vi "Read CamName and ImageType.vi"(8 "error in (no error)":errorcluster, 11 "IMAQdx Cam in":refnum<class "IMAQdx Cam.lvclass">) -> (0 "error out":errorcluster, 1 "Camera":T1, 2 "Image Type":T2 items=["Grayscale (U8)", "Grayscale (I16)", "Grayscale (SGL)", "Complex (CSG)", "RGB (U32)", "HSL (U32)", "RGB (U64)", "Grayscale (U16)"], 3 "IMAQdx Cam out":refnum<class "IMAQdx Cam.lvclass">)   [LabVIEW 2009, in "IMAQdx Cam.lvclass"]
uses:
  IMAQdx Cam.lvclass
  <vilib>/userDefined/High Color/IMAQdx.ctl
  IMAQdx Cam.lvclass/IMAQdx Cam.ctl
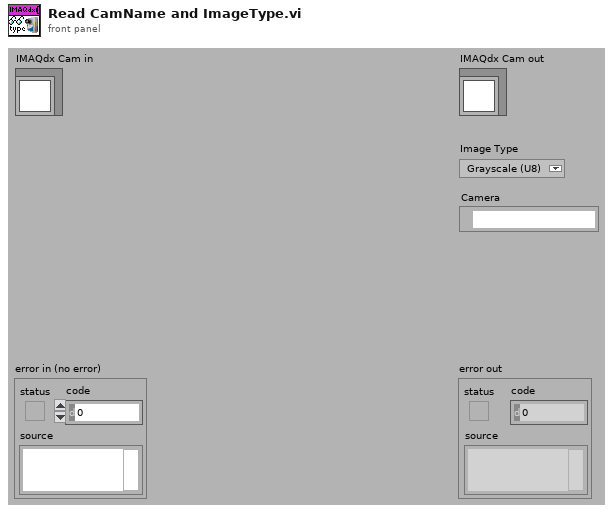
[diagram p1: front panel]
types:
  T1 = typedef "IMAQdx.ctl" = refnum<k21>
  T2 = typedef "Image Type" = u32
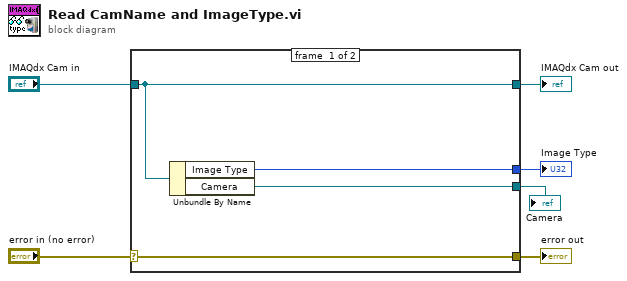
[diagram p0: block diagram]
diagram:
  n1 = case shown="No Error" "error in (no error)" {
    selector: "error in (no error)" -> [w10 w11]
    tunnel: [w10 w11] -> w5
    tunnel: [w9 w12] -> w3
    tunnel: "IMAQdx Cam in" -> [w9 w12]
    tunnel: [w8 _] -> w2
    tunnel: [w7 _] -> w1
    frame #0 {
      n2 = Unbundle By Name(w9) -> ("Image Type"=w8:T2, "Camera"=w7:T1)
    }
    frame #1 {
    }
  }
  "error out" <- w5
  "IMAQdx Cam out" <- w3
  "Image Type" <- w2
  "Camera" <- w1
